vi "AcqBdcst.vi"(8 "error in (no error)":errorcluster, 10 "Acquisition":T1 {"SampleMode" items=["Real Time", "Equivalent Time"]}, 11 "Module":refnum<class "ModuleAdmin.lvclass">) -> (0 "error out":errorcluster, 3 "Module":refnum<class "ModuleAdmin.lvclass">)   [LabVIEW 2014, in "DigitizerPlugins.lvlib" / "DigitizerBase.lvclass"]
uses:
  DigitizerBase.lvclass
  <userlib>/NIST/ModuleAdminLib/ModuleAdmin/ModuleAdmin.lvclass
  Typedefs/Acquisition.ctl
  DigitizerModule/Protected/clEventType.ctl
  DigitizerModule/DigitizerModule.lvlib
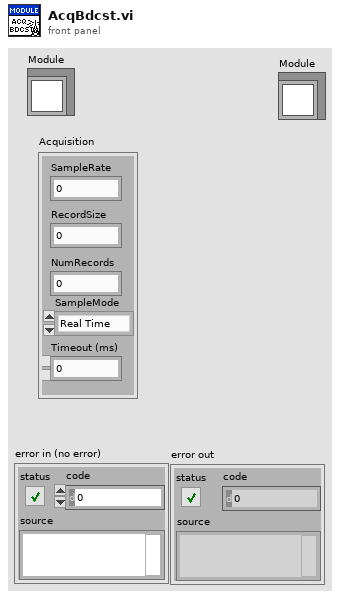
[diagram p1: front panel]
types:
  T1 = typedef "DigitizerPlugins.lvlib/DigitizerBase.lvclass/Acquisition.ctl" = cluster{"SampleRate":dbl, "RecordSize":i32, "NumRecords":i32, "SampleMode":i32, "Timeout (ms)":i32}
  T2 = typedef "DigitizerModule.lvlib/clEventType.ctl" = cluster{"ModuleID":i32, "Data":variant}
  T3 = typedef "DigitizerModule.lvlib/clBroadcastEvents.ctl" = cluster{"DidInit":refnum<user-event>, "StatusUpdate":refnum<user-event>, "ErrorReport":refnum<user-event>, "DidStop":refnum<user-event>, "PathToINI":refnum<user-event>, "Channels":refnum<user-event>, "Acq":refnum<user-event>, "Trigger":refnum<user-event>, "Waveforms":refnum<user-event>}
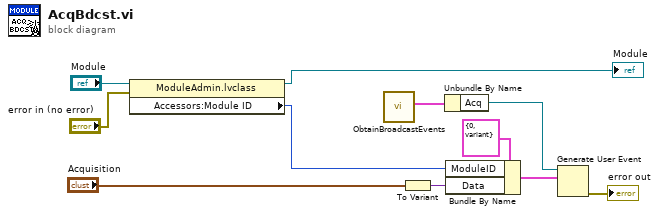
[diagram p0: block diagram]
diagram:
  n1 = property class="ModuleAdmin.lvclass"(reference="Module", error in="error in (no error)") -> (reference out=→"Module":refnum<class "ModuleAdmin.lvclass">, "Accessors:Module ID"=w4:i32)  [unwired: 1 out]
  n2 = call "ObtainBroadcastEvents.vi"() -> ("clDigitizerBdcstEvents"=w11:T3)  [unwired: 10 in, 1 out]
  n3 = To Variant(anything="Acquisition") -> (Variant=w8:variant)
  n4 = Unbundle By Name(w11) -> ("Acq"=w10:refnum<user-event>)
  n5 = Bundle By Name(cluster=T2 {"ModuleID"=0, "Data"=variant} ("clBroadcast"), "ModuleID"=w4, "Data"=w8) -> (w7:T2)
  n6 = Generate User Event(user event=w10, event data cluster=w7) -> (error out=→"error out":errorcluster)  [unwired: 2 in, 1 out]
